vi "LIA 5783 Getting Started FPGA.vi"() -> ()   [LabVIEW 2018]
doc: "Example Description:\nThis example acquires records of analog input data and generates analog output data from the NI 5783 adapter module. For the analog input, it allows the user to select an AI channel, trigger type, and record size. For the analog output, it allows the user to select AO channel, waveform signal type, frequency, amplitude, and sampling information. This VI is compiled for all FPGA targets by default.\n\nRunning the VI:\nThis VI must be run from the NI 5783 - Getting Started (Host).vi. Refer to the host VI documentation for steps regarding running and configuring the FPGA VI. \n\nExecution Steps:\nRefer to the Block Diagram of this VI for execution comments."
uses:
  <vilib>/eio/EIONode/EIONode.xnode
  <vilib>/Platform/TimedLoop/XDataNode/XDataNode.xnode
  <vilib>/Platform/TimedLoop/XDataNode/nitl_modes.ctl
  <vilib>/Platform/TimedLoop/XDataNode/XDNodeRunTimeDep.lvlib
  <vilib>/Platform/TimedLoop/XDataNode/wakeup.ctl
  <vilib>/Platform/TimedLoop/XDataNode/timing_clust.ctl
  <vilib>/rvi/DataTransferAndStorage/Container/XNode/niFpgaContainer.xnode
  <vilib>/rvi/eio/common/nirviEmuTemplateMethod_errors.vi
  <instrlib>/_niInstr/Streaming/v1/FPGA/niInstr Streaming v1 FPGA.lvlib
  <vilib>/rvi/Memory/Memory_Emulation/nirvimemoryEmulation.vi
  <vilib>/rvi/Memory/Memory_Emulation/nirvimemoryFastEmulation.vi
  <vilib>/rvi/interface/RandomDataEmulation/nirviRandomDataFpgaMultiElementTemplate.vi
  <instrlib>/_niInstr/Basic Elements/v1/FPGA/niInstr Basic Elements v1 FPGA.lvlib
  <instrlib>/_niInstr/Data Trigger/v1/FPGA/niInstr Data Trigger v1 FPGA.lvlib
  <instrlib>/_niInstr/Data Trigger/v1/FPGA/Private/Trigger/Level I16xNspc.vi
  <vilib>/rvi/interface/RandomDataEmulation/nirviRandomDataFpgaReadWriteTemplate.vi
  Program Files (x86)/National Instruments/LabVIEW 2017/examples/FlexRIO/IO Modules/NI 5783/NI 5783 - Getting Started/Controls/AI Trigger Type.ctl
  Program Files (x86)/National Instruments/LabVIEW 2017/examples/FlexRIO/IO Modules/NI 5783/NI 5783 - Getting Started/Controls/AO Channel.ctl
  <instrlib>/_niInstr/Streaming/v1/Common/Stream State.ctl
  <instrlib>/_niInstr/Streaming/v1/Common/niInstr Streaming v1 Common.lvlib
  <instrlib>/_niInstr/Data Trigger/v1/Shared/Public/Level Configuration Trigger When.ctl
  <instrlib>/_niInstr/Data Trigger/v1/Shared/niInstr Data Trigger v1 Shared.lvlib
  <instrlib>/_niInstr/Data Trigger/v1/Shared/Public/Level Configuration I16.ctl
panel:
  in  "channel index":i32
  in  "Trigger Configuration":T1
  out "IO Module\\User Command Return Valid":bool
  out "IO Module\\User Command Return":u32
  out "IO Module\\User Command Error":u16
  in  "IO Module\\User Command Arg 1":u32
  in  "IO Module\\User Command Arg 0":u32
  out "IO Module\\User Command Ready":bool
  in  "IO Module\\User Command Valid":bool
  in  "IO Module\\User Command":u32
  out "IO Module\\User Error":u32
  in  "stream.request state 2":T3
  in  "stream.num samples 2":u64
  out "stream.metadata 2":u64
  out "stream.samples transferred 2":u64
  out "stream.state 2":T3
  in  "stream.num samples 1":u64
  out "stream.state 1":T3
  out "stream.samples transferred 1":u64
  in  "stream.request state 1":T3
  out "stream.metadata 1":u64
  in  "stream.num samples 0":u64
  out "stream.state 0":T3
  out "stream.samples transferred 0":u64
  in  "stream.request state 0":T3
  out "stream.metadata 0":u64
  in  "AO Channel":T4
  in  "Trigger Type":T5
  out "IO Module\\InitDone":bool
  # "Refer to the Block Diagram of this VI for execution comments."
  # "For other instructions, select Help>>Show Context Help and move the cursor over the VI icon to display help for this VI."
  # "Analog Input"
  # "Analog Output"
  # "Resource Configuration"
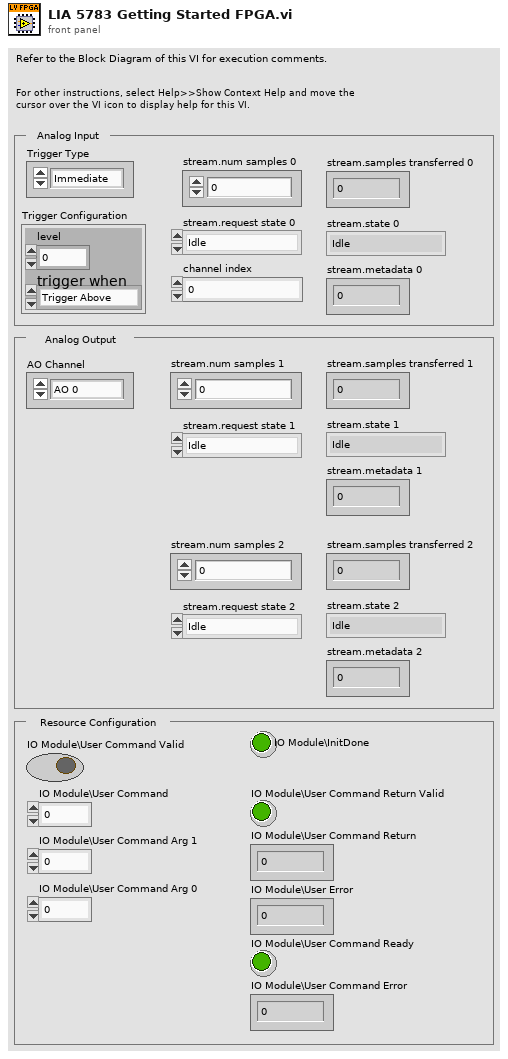
[diagram p1: front panel]
types:
  T1 = typedef "niInstr Data Trigger v1 Shared.lvlib/Level Configuration I16.ctl" = cluster{"level":i16, "trigger when":T2}
  T2 = typedef "niInstr Data Trigger v1 Shared.lvlib/Level Configuration Trigger When.ctl" = enum8{"Trigger Above", "Trigger Below"}
  T3 = typedef "niInstr Streaming v1 Common.lvlib/Stream State.ctl" = enum8{"Idle", "Finite Transfer", "Continuous", "Done", "Error", "Not Ready", "Cancel"}
  T4 = typedef "AO Channel.ctl" = enum8{"AO 0", "AO 1", "AO 2", "AO 3", "AO 0, AO 1, AO 2, AO 3", "None"}
  T5 = typedef "AI Trigger Type.ctl" = enum8{"Immediate", "Data Trigger", "TRIG input"}
  T6 = typedef "XDNodeRunTimeDep.lvlib/timing_clust.ctl" = cluster{"Expected End [f-1]":u64, "Actual End [f-1]":u64, "Finished Late? [f-1]":bool, "Expected End [i-1]":u64, "Actual End [i-1]":u64, "Finished Late? [i-1]":bool, "Expected Start [i]":u64, "Actual Start [i]":u64, "Expected Start [f]":u64, "Actual Start [f]":u64, "Source Name":string, "Structure Name":string, "Period":i64, "Deadline":i64, "Offset":i64, "Start":i64, "Priority":i32, "Timeout":i32, "Mode":T7, "Wakeup Reason":T8, "Error":errorcluster, "Source Type":string, "Secondary Source Type":string, "Global End Time":u64, "Global Start Time":u64, "Frame Duration":u64, "Iteration Duration":u64, "Assigned CPU":i32, "I/O Scan Engine Mode":u32}
  T7 = typedef "XDNodeRunTimeDep.lvlib/nitl_modes.ctl" = enum32{"No Change", "Process missed periods, maintain original phase", "Discard missed periods, maintain original phase", "Process missed periods, ignore original phase", "Discard missed periods, ignore original phase"}
  T8 = typedef "XDNodeRunTimeDep.lvlib/wakeup.ctl" = enum32{"Normal", "Aborted", "Asynchronous wakeup", "Timing source error", "Timed loop error", "Timeout"}
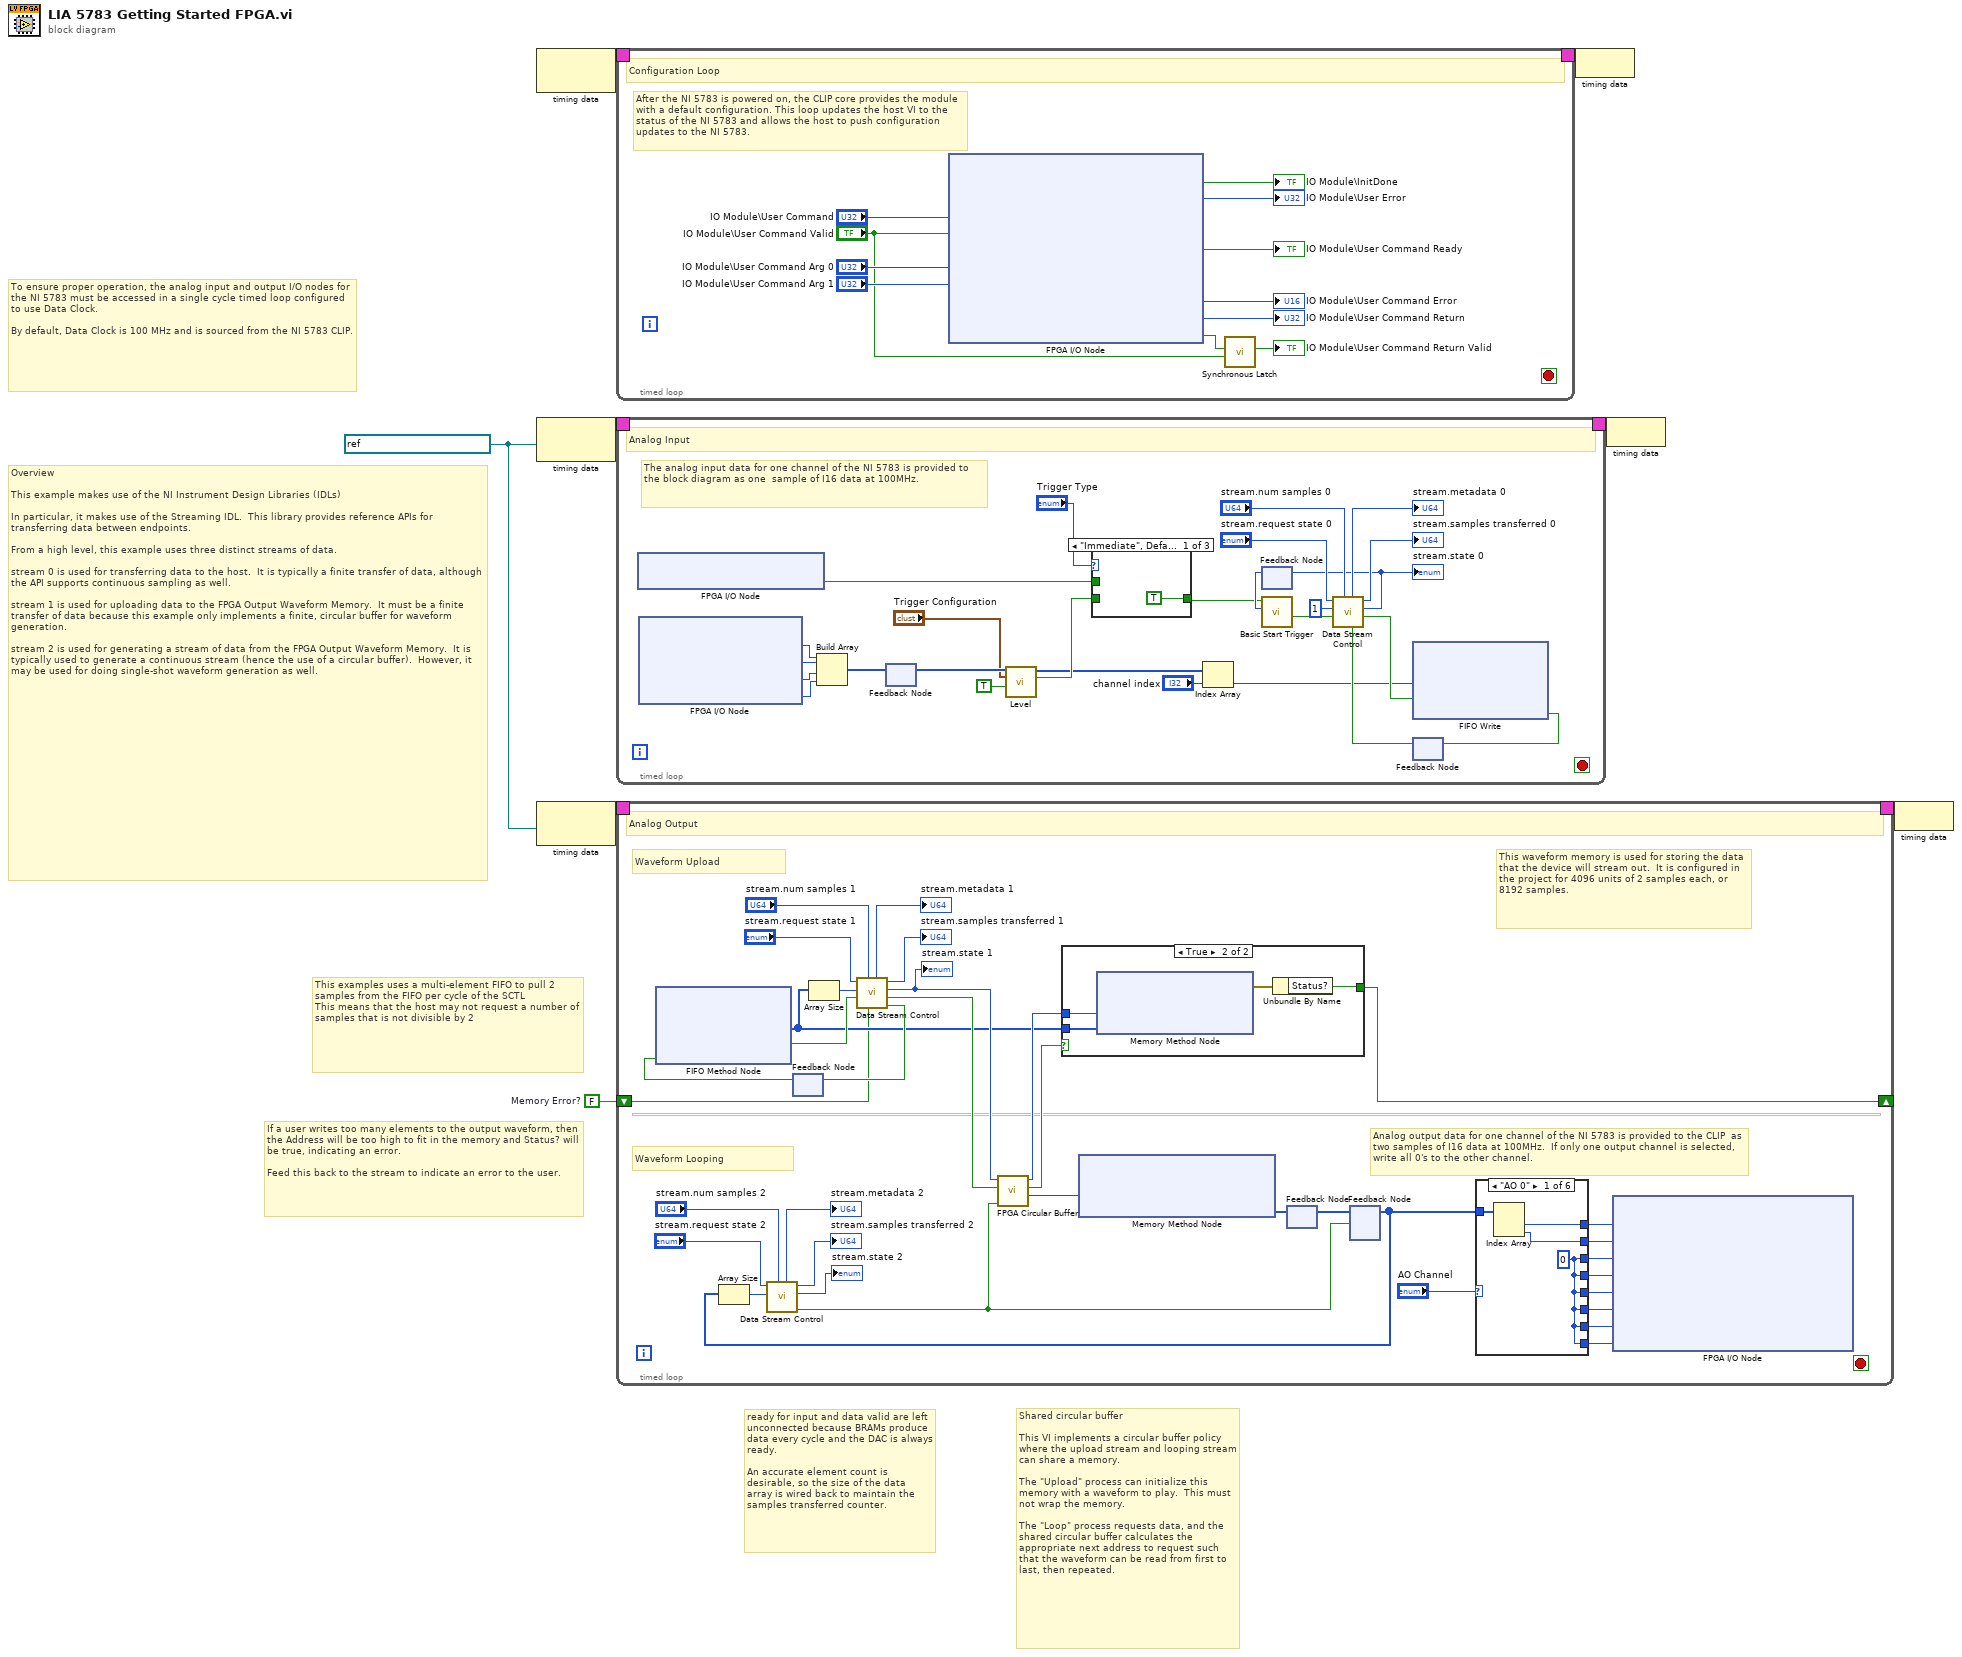
[diagram p0: block diagram]
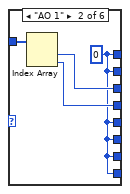
[diagram p3: hidden frame]
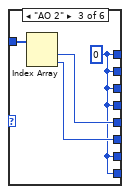
[diagram p4: hidden frame]
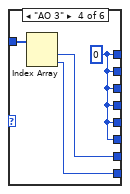
[diagram p5: hidden frame]
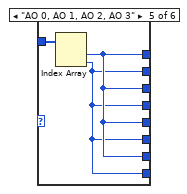
[diagram p6: hidden frame]
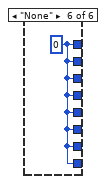
[diagram p7: hidden frame]
diagram:
  w1 = FALSE  # Memory Error?
  w4 = refnum<k21> "IO Module\\Data Clock" ("Source Name")
  # "If a user writes too many elements to the output waveform, then the Address will be too high to fit in the memory and Status? will be true, indicating an error.\n\nFeed this back to the stream to indicate an error to the user."
  # "ready for input and data valid are left unconnected because BRAMs produce data every cycle and the DAC is always ready.\n\nAn accurate element count is desirable, so the size of the data array is wired back to maintain the samples transferred counter."
  # "Overview\n\nThis example makes use of the NI Instrument Design Libraries (IDLs)\n\nIn particular, it makes use of the Streaming IDL.  This library provides reference APIs for transferring data between endpoints.\n\nFrom a high level, this example uses three distinct streams of data.\n\nstream 0 is used for transferring data to the host.  It is typically a finite transfer of data, although the API supports continuous sampling as well.\n\nstream 1 is used for uploading data to the FPGA Output Waveform Memory.  It must be a finite transfer of data because this example only implements a finite, circular buffer for waveform generation.\n\nstream 2 is used for generating a stream of data from the FPGA Output Waveform Memory.  It is typically used to generate a continuous stream (hence the use of a circular buffer).  However, it may be used for doing single-shot waveform generation as well."
  # "Shared circular buffer\n\nThis VI implements a circular buffer policy where the upload stream and looping stream can share a memory.\n\nThe \"Upload\" process can initialize this memory with a waveform to play.  This must not wrap the memory.  \n\nThe \"Loop\" process requests data, and the shared circular buffer calculates the appropriate next address to request such that the waveform can be read from first to last, then repeated."
  # "This examples uses a multi-element FIFO to pull 2 samples from the FIFO per cycle of the SCTL\nThis means that the host may not request a number of samples that is not divisible by 2"
  # "To ensure proper operation, the analog input and output I/O nodes for the NI 5783 must be accessed in a single cycle timed loop configured to use Data Clock. \n\nBy default, Data Clock is 100 MHz and is sourced from the NI 5783 CLIP."
  n1 = node-c288() -> (w3:T6)  [unwired: 1 in]
  n2 = node-c288(w4) -> (w8:T6)
  n3 = node-c288 ("Input Node")(w4) -> (w6:T6)
  n4 = timed-loop {
    timing: w3 -> [_]
    timing-out: [_] -> w2
    stop <- _ stop-if-true
    # "After the NI 5783 is powered on, the CLIP core provides the module with a default configuration. This loop updates the host VI to the status of the NI 5783 and allows the host to push configuration updates to the NI 5783."
    # "Configuration Loop"
    n5 = xnode "FPGA I/O Node"("IO Module\\User Command"="IO Module\\User Command", "IO Module\\User Command Valid"="IO Module\\User Command Valid", "IO Module\\User Command Arg 0"="IO Module\\User Command Arg 0", "IO Module\\User Command Arg 1"="IO Module\\User Command Arg 1") -> ("IO Module\\InitDone"=→"IO Module\\InitDone":bool, "IO Module\\Clip Error Code"=→"IO Module\\User Error":u32, "IO Module\\User Command Ready"=→"IO Module\\User Command Ready":bool, "IO Module\\User Command Error"=→"IO Module\\User Command Error":u16, "IO Module\\User Command Return"=→"IO Module\\User Command Return":u32, "IO Module\\User Command Return Valid"=w10:bool)  [unwired: 10 in, 10 out]
    n6 = call <instrlib>:"Synchronous Latch.vi"("clear"="IO Module\\User Command Valid", "set"=w10) -> ("out"=→"IO Module\\User Command Return Valid":bool)  [unwired: 9 in]
  }
  n7 = timed-loop {
    timing: w8 -> [_]
    timing-out: [_] -> w7
    stop <- _ stop-if-true
    # "The analog input data for one channel of the NI 5783 is provided to the block diagram as one  sample of I16 data at 100MHz."
    # "Analog Input"
    n8 = xnode "FPGA I/O Node"() -> ("IO Module\\Trigger Rd Data"=w30:bool)  [unwired: 1 in, 1 out]
    n9 = xnode "FPGA I/O Node"() -> ("IO Module\\AI 0 Data N"=w35:i16, "IO Module\\AI 1 Data N"=w34:i16, "IO Module\\AI 2 Data N"=w33:i16, "IO Module\\AI 3 Data N"=w32:i16)  [unwired: 4 in, 4 out]
    n10 = Build Array(w35, w34, w33, w32) -> (w31:i16[])
    n11 = feedback-in #1(w31) -> ()
    n12 = feedback #1() -> (w29:i16[])  [unwired: 1 in]
    n13 = call-poly <instrlib>:"Level.vi"("data in"=w29, "configuration"="Trigger Configuration", "input valid"=TRUE) -> ("data out"=w24:i16[], "trigger"=w28:bool)  [unwired: 7 in, 4 out]
    n14 = case shown="\"Immediate\", Default" "Trigger Type" {
      tunnel: w28 -> [_ w49 _]
      tunnel: [TRUE ("Trigger") w49 w50] -> w36
      tunnel: w30 -> [_ _ w50]
      frame "Immediate", Default {
      }
      frame "Data Trigger" {
      }
      frame "TRIG input" {
      }
    }
    n15 = Index Array(array=w24, index="channel index") -> (element=w23:i16)
    n16 = feedback #2() -> (w42:T3)  [unwired: 1 in]
    n17 = call <instrlib>:"Basic Start Trigger.vi"("stream.state"=w42, "start trigger"=w36) -> ("data valid"=w43:bool)  [unwired: 9 in]
    n18 = feedback #3() -> (w38:bool)  [unwired: 1 in]
    n19 = call <instrlib>:"Data Stream Control.vi"("ready for input?"=w38, "stream.num samples 0"="stream.num samples 0", "data valid"=w43, "element count"=u16 1, "stream.request state 0"="stream.request state 0") -> ("send data"=w40:bool, "stream.state 0"=w41:T3, "stream.samples transferred 0"=→"stream.samples transferred 0":u64, "stream.metadata 0"=→"stream.metadata 0":u64)  [unwired: 2 in, 1 out]
    "stream.state 0" <- w41
    n20 = feedback-in #2(w41) -> ()
    n21 = xnode ("FIFO Write")("Element"=w23, "Input Valid"=w40) -> ("Ready for Input"=w39:bool)  [unwired: 1 in, 1 out]
    n22 = feedback-in #3(w39) -> ()
  }
  n23 = timed-loop {
    timing: w6 -> [_]
    timing-out: [_] -> w5
    shift-right: [w56] -> _
    shift-left: w1 -> [w57]
    stop <- _ stop-if-true
    # "This waveform memory is used for storing the data that the device will stream out.  It is configured in the project for 4096 units of 2 samples each, or 8192 samples."
    # "Waveform Upload"
    # "Waveform Looping"
    # "Analog output data for one channel of the NI 5783 is provided to the CLIP  as two samples of I16 data at 100MHz.  If only one output channel is selected, write all 0's to the other channel."
    # "Analog Output"
    n24 = feedback #4() -> (w72:bool)  [unwired: 1 in]
    n25 = xnode ("FIFO Method Node")("Ready for Output"=w72) -> ("Element"=w61:i16[], "Output Valid"=w74:bool)  [unwired: 1 in, 1 out]
    n26 = Array Size(array=w61) -> (size(s)=w75:i32)
    n27 = call <instrlib>:"Data Stream Control.vi"("force error"=w57, "stream.num samples 0"="stream.num samples 1", "data valid"=w74, "element count"=w75, "stream.request state 0"="stream.request state 1") -> ("request data"=w73:bool, "send data"=w64:bool, "stream.state 0"=w66:T3, "stream.samples transferred 0"=→"stream.samples transferred 1":u64, "stream.metadata 0"=→"stream.metadata 1":u64)  [unwired: 2 in]
    "stream.state 1" <- w66
    n28 = feedback-in #4(w73) -> ()
    n29 = feedback #5() -> (w54:i16[])  [unwired: 1 in]
    n30 = feedback #6() -> (w53:i16[])  [unwired: 1 in]
    n31 = Array Size(array=w53) -> (size(s)=w55:i32)
    n32 = call <instrlib>:"Data Stream Control.vi"("stream.num samples 0"="stream.num samples 2", "element count"=w55, "stream.request state 0"="stream.request state 2") -> ("request data"=w59:bool, "stream.state 0"=→"stream.state 2":T3, "stream.samples transferred 0"=→"stream.samples transferred 2":u64, "stream.metadata 0"=→"stream.metadata 2":u64)  [unwired: 4 in, 1 out]
    n33 = call "FPGA Circular Buffer.vi"("request data"=w59, "send data"=w64, "stream.state 0"=w66) -> ("Read Pointer"=w58:u32, "send data out"=w60:bool, "Write Pointer"=w62:u32)  [unwired: 6 in]
    n34 = case shown="True" w60 {
      tunnel: w62 -> [_ w91]
      tunnel: w61 -> [_ w90]
      tunnel: [_ w88] -> w56
      frame False {
      }
      frame True {
        n35 = xnode ("Memory Method Node")("Address"=w91, "Data"=w90) -> ("error out"=w89:errorcluster)  [unwired: 2 in, 1 out]
        n36 = Unbundle By Name(w89) -> ("Status?"=w88:bool)
      }
    }
    n37 = xnode ("Memory Method Node")("Address"=w58) -> ("Data"=w63:i16[])  [unwired: 1 in, 1 out]
    n38 = feedback-in #5(w63) -> ()
    n39 = feedback-in #6(w54, w59) -> ()
    n40 = case shown="\"AO 0\"" "AO Channel" {
      tunnel: w53 -> [w95 w99 w103 w107 w110 _]
      tunnel: [w92 w96 w101 w104 w109 w111] -> w87
      tunnel: [w93 w96 w100 w104 w108 w111] -> w86
      tunnel: [w92 w96 w100 w105 w108 w111] -> w85
      tunnel: [w92 w96 w102 w104 w108 w111] -> w84
      tunnel: [w92 w96 w100 w106 w109 w111] -> w83
      tunnel: [w92 w97 w100 w104 w108 w111] -> w82
      tunnel: [w92 w98 w100 w104 w109 w111] -> w81
      tunnel: [w94 w96 w100 w104 w109 w111] -> w80
      frame "AO 0" {
        w92 = i16 0 ("Data")
        n41 = Index Array(array=w95) -> (element #1=w94:i16, element #2=w93:i16)  [unwired: 2 in]
      }
      frame "AO 1" {
        w96 = i16 0 ("I16")
        n42 = Index Array(array=w99) -> (element #1=w98:i16, element #2=w97:i16)  [unwired: 2 in]
      }
      frame "AO 2" {
        w100 = i16 0 ("I16")
        n43 = Index Array(array=w103) -> (element #1=w101:i16, element #2=w102:i16)  [unwired: 2 in]
      }
      frame "AO 3" {
        w104 = i16 0 ("I16")
        n44 = Index Array(array=w107) -> (element #1=w106:i16, element #2=w105:i16)  [unwired: 2 in]
      }
      frame "AO 0, AO 1, AO 2, AO 3" {
        n45 = Index Array(array=w110) -> (element #1=w109:i16, element #2=w108:i16)  [unwired: 2 in]
      }
      frame "None" {
        w111 = i16 0 ("I16")
      }
    }
    n46 = xnode "FPGA I/O Node"("IO Module\\AO 0 Data N-1 Data Clock"=w80, "IO Module\\AO 0 Data N Data Clock"=w86, "IO Module\\AO 1 Data N-1 Data Clock"=w81, "IO Module\\AO 1 Data N Data Clock"=w82, "IO Module\\AO 2 Data N-1 Data Clock"=w87, "IO Module\\AO 2 Data N Data Clock"=w84, "IO Module\\AO 3 Data N-1 Data Clock"=w83, "IO Module\\AO 3 Data N Data Clock"=w85) -> ()  [unwired: 8 in, 8 out]
  }
  n47 = node-c288(w2) -> ()
  n48 = node-c288(w7) -> ()
  n49 = node-c288(w5) -> ()
